vi "LakeShore218_Global.vi"() -> ()   [LabVIEW 2019]
panel:
  out "LS218_02_T8":dbl
  out "LS218_02_T7":dbl
  out "LS218_02_T6":dbl
  out "LS218_02_T5":dbl
  out "LS218_02_T4":dbl
  out "LS218_02_T3":dbl
  out "LS218_02_T2":dbl
  out "LS218_02_ST":u32(colorbox)
  out "LS218_02_T1":dbl
  out "LS218_01_T8":dbl
  out "LS218_01_T7":dbl
  out "LS218_01_T6":dbl
  out "LS218_01_T5":dbl
  out "LS218_01_T4":dbl
  out "LS218_01_T3":dbl
  out "LS218_01_T2":dbl
  out "LS218_01_ST":u32(colorbox)
  out "LS218_01_T1":dbl
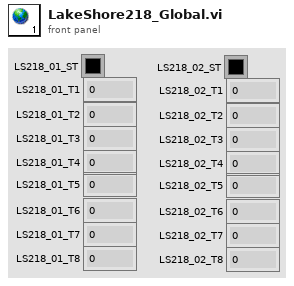
[diagram p1: front panel]
diagram:
